vi "Get Simulated Classes.vi"(8 "error in (no error)":errorcluster, 9 "sim servo freq":dbl=30.0, 10 "sim force freq":dbl=30.0, 11 "sim cam freq":dbl=30.0) -> (0 "error out":errorcluster, 1 "sim switch":refnum<class "Simulated Switch.lvclass">, 2 "sim servo":refnum<class "Simulated Servo.lvclass">, 3 "sim fs":refnum<class "Simulated Force Sensor.lvclass">, 5 "sim cam":refnum<class "Simulated Camera.lvclass">)   [LabVIEW 2020]
uses:
  Actuators/Switches/Simulated Switch/Simulated Switch.lvclass
  Actuators/Servos/Simulated Servo/Simulated Servo.lvclass
  C:/Users/jharw/Documents/1 Folder to Rule them All/UMD/Inflation-Apparatus/src/Hardware/General Hardware.lvclass
  Sensors/Force Sensors/Simulated Force Sensor/Simulated Force Sensor.lvclass
  Sensors/Cameras/Simulated Camera/Simulated Camera.lvclass
  General Hardware.lvclass/General Hardware.ctl
  General Hardware.lvclass
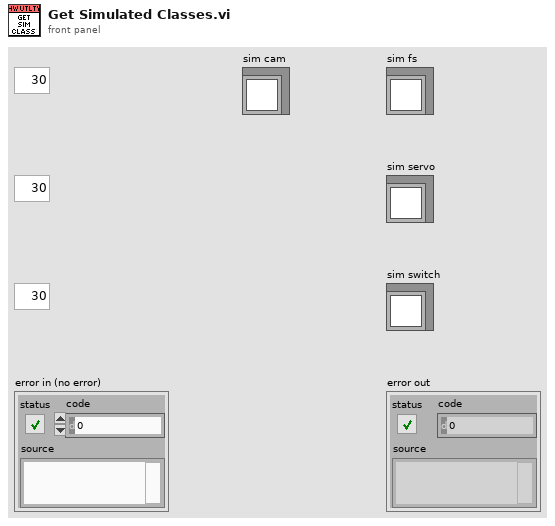
[diagram p1: front panel]
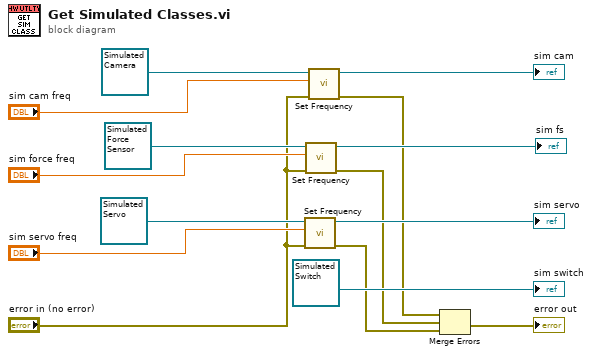
[diagram p0: block diagram]
diagram:
  n1 = call "Set Frequency.vi"("error in (no error)"="error in (no error)", "frequency (Hz)"="sim servo freq", "General Hardware in"=refnum<class "Simulated Servo.lvclass"> refnum ("Simulated Servo.lvclass")) -> ("error out"=w4:errorcluster, "General Hardware out"=→"sim servo":refnum<class "Simulated Servo.lvclass">)  [unwired: 7 in]
  n2 = call "Set Frequency.vi"("error in (no error)"="error in (no error)", "frequency (Hz)"="sim force freq", "General Hardware in"=refnum<class "Simulated Force Sensor.lvclass"> refnum ("Simulated Force Sensor.lvclass")) -> ("error out"=w3:errorcluster, "General Hardware out"=→"sim fs":refnum<class "Simulated Force Sensor.lvclass">)  [unwired: 7 in]
  n3 = call "Set Frequency.vi"("error in (no error)"="error in (no error)", "frequency (Hz)"="sim cam freq", "General Hardware in"=refnum<class "Simulated Camera.lvclass"> refnum ("Simulated Camera.lvclass")) -> ("error out"=w2:errorcluster, "General Hardware out"=→"sim cam":refnum<class "Simulated Camera.lvclass">)  [unwired: 7 in]
  n4 = Merge Errors(w2, w3, w4) -> (→"error out":errorcluster)
  "sim switch" <- refnum<class "Simulated Switch.lvclass"> refnum ("Simulated Switch.lvclass")
